vi "Configure PRACH Enable All Results.vi"(8 "error in (no error)":errorcluster, 9 "Enable All Results":bool[](array[boolean]), 10 "Instance (1)":T1=1, 11 "VISA resource name":refnum<visa-resource-name>) -> (0 "error out":errorcluster, 3 "VISA resource name out":refnum<visa-resource-name>)   [LabVIEW 2020, in "Rohde&Schwarz CMWXP NR FR1 Measurement.lvlib"]
doc: "Enables or disables the evaluation of results in the PRACH measurement.\n\nAttribute:\nRSCMWXPNRFR1M_ATTR_PRACH_ENABLE_ALL_RESULTS\n\nRemote-control command:\nCONFigure:NRSub:MEAS<i>:PRACh:RESult[:ALL]"
uses:
  <instrlib>/Rohde&Schwarz CMWXP NR FR1 Measurement/Rohde&Schwarz CMWXP NR FR1 Measurement.lvlib
  <instrlib>/Rohde&Schwarz CMWXP NR FR1 Measurement/Private/_Instance.ctl
  <instrlib>/Rohde&Schwarz CMWXP NR FR1 Measurement/Private/rsidr_core.llb/rsidr_core.lvlib
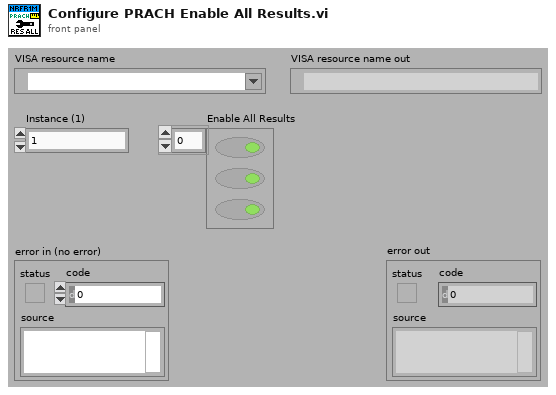
[diagram p1: front panel]
types:
  T1 = typedef "Rohde&Schwarz CMWXP NR FR1 Measurement.lvlib/_Instance.ctl" = i32
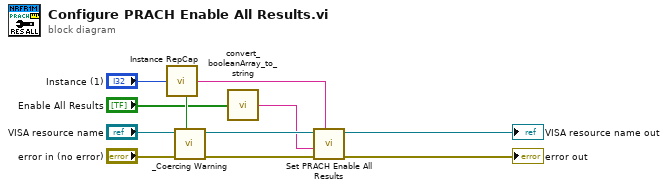
[diagram p0: block diagram]
diagram:
  n1 = call <instrlib>:"Instance RepCap.vi"("Instance In"="Instance (1)") -> ("In Range?"=w3:bool, "RepCap Identifier Out"=w4:string)  [unwired: 1 in]
  n2 = call <instrlib>:"_Coercing Warning.vi"("In Range?"=w3, "error in (no error)"="error in (no error)", "VISA resource name"="VISA resource name") -> ("error out"=w7:errorcluster, "VISA resource name out"=w6:refnum<visa-resource-name>)  [unwired: 7 in]
  n3 = call <instrlib>:"convert_booleanArray_to_string.vi"("Boolean array in"="Enable All Results") -> ("string out"=w2:string)  [unwired: 4 in]
  n4 = call "Set PRACH Enable All Results"("Repeated Capabilities"=w4, "error in (no error)"=w7, "PRACH Enable All Results ()"=w2, "instrument handle"=w6) -> ("error out"=→"error out":errorcluster, "instrument handle out"=→"VISA resource name out":refnum<visa-resource-name>)  [unwired: 6 in]
